vi "DAQ.44xx.Get Product Type from Device.vi"(8 "error in (no error)":errorcluster, 11 "DAQmx Device Name":tag) -> (0 "error out":errorcluster, 2 "DAQ Type":T1, 3 "DevIsSimulated":bool)   [LabVIEW 2019, in "Instrument.DAQ.lvclass"]
uses:
  Instrument.DAQ.lvclass
  Typedefs/DAQ.Type--enum.ctl
  <resource>/objmgr/daqmx.rc
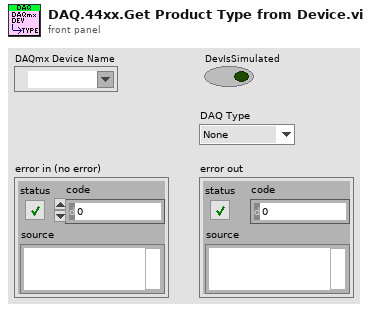
[diagram p1: front panel]
types:
  T1 = typedef "Instrument.DAQ.lvclass/DAQ.Type--enum.ctl" = enum16{"None", "USB-4431", "PXI-446x"}
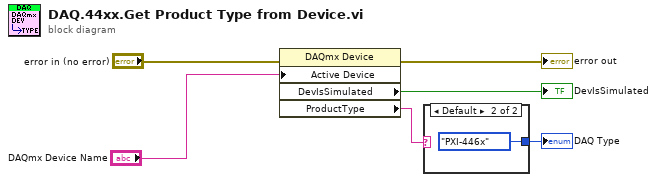
[diagram p0: block diagram]
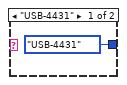
[diagram p2: hidden frame]
diagram:
  n1 = property class="DAQmx Device"(error in="error in (no error)", "Active Device"="DAQmx Device Name") -> (error out=→"error out":errorcluster, "DevIsSimulated"=→"DevIsSimulated":bool, "ProductType"=w5:string)  [unwired: 1 in, 1 out]
  n2 = case shown="Default" w5 {
    tunnel: [DAQ.Type--enum."USB-4431" ("DAQ Type") DAQ.Type--enum."PXI-446x" ("DAQ Type")] -> w3
    frame "USB-4431" {
    }
    frame Default {
    }
  }
  "DAQ Type" <- w3
